vi "Read Data Value.vi"(8 "error in (no error)":errorcluster, 11 "ValueReferenceTransport In":refnum<class "ValueReferenceTransport.lvclass">) -> (0 "error out":errorcluster, 1 "Publication Time":timestamp, 2 "Data":variant)   [LabVIEW 2017, in "Transport.lvlib" / "ValueReferenceTransport.lvclass"]
uses:
  ValueReferenceTransport.lvclass
  ValueReferenceTransport.lvclass/ValueReferenceTransport.ctl
  <vilib>/Utility/error.llb/Error Cluster From Error Code.vi
  <vilib>/ErrorRing/Error Ring.xnode
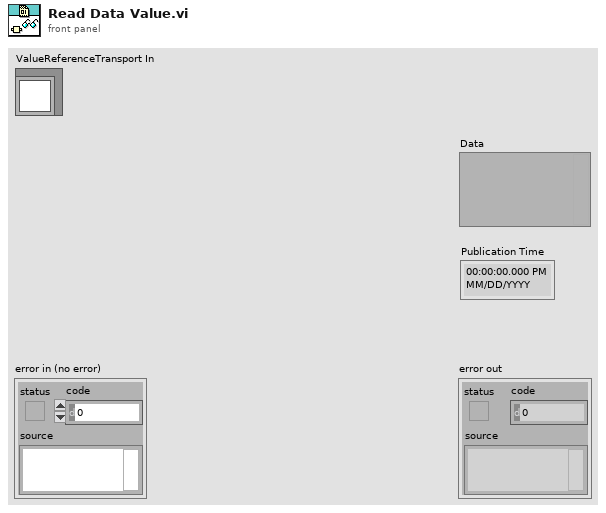
[diagram p1: front panel]
types:
  T1 = cluster{"Data":variant, "Publication Time":timestamp}
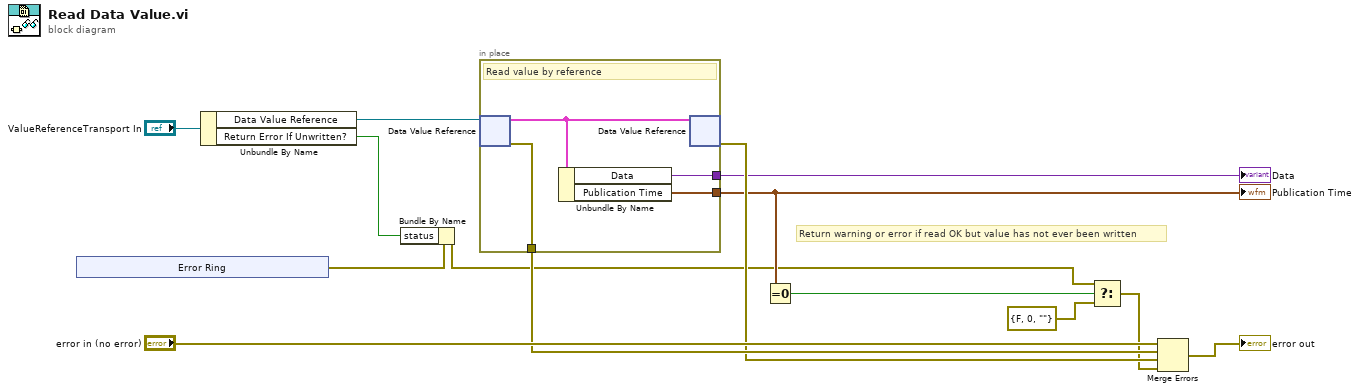
[diagram p0: block diagram]
diagram:
  # "Return warning or error if read OK but value has not ever been written"
  n1 = xnode "Error Ring"() -> ("error out"=w4:errorcluster)
  n2 = Unbundle By Name("ValueReferenceTransport In") -> ("Data Value Reference"=w12:refnum<data-value>, "Return Error If Unwritten?"=w1:bool)
  n3 = Bundle By Name(cluster=w4, "status"=w1) -> (w2:errorcluster)
  n4 = in-place {
    in-place-border: [w17] -> w8
    in-place-border: [w16] -> w7
    in-place-border: [w15] -> w10
    # "Read value by reference"
    n5 = in-place-dvr #1(w12) -> (w18:T1, w15:errorcluster)
    n6 = Unbundle By Name(w18) -> ("Data"=w17:variant, "Publication Time"=w16:timestamp)
    n7 = in-place-dvr #1(w18) -> (w9:errorcluster)  [unwired: 1 out]
  }
  "Data" <- w8
  "Publication Time" <- w7
  n8 = Equal To 0?(x=w7) -> (x = 0?=w6:bool)
  n9 = Select(t=w2, s=w6, f=errorcluster {"status"=FALSE, "code"=0, "source"=""}) -> (s? t:f=w5:errorcluster)
  n10 = Merge Errors("error in (no error)", w10, w9, w5) -> (→"error out":errorcluster)
